vi "Signal List Keys.vi"(8 "error in":errorcluster, 11 "PRM in":refnum<class "PRM.lvclass">) -> (0 "error out":errorcluster, 2 "CFG Signal Headers":string[](array[string]), 3 "PRM out":refnum<class "PRM.lvclass">)   [LabVIEW 2019, in "PRM.lvlib" / "PRM.lvclass"]
uses:
  Library/PRM.lvclass
  Custom Controls/Signal List Keys.ctl
  builds/Instruments/Instruments.lvlibp/Library/Instruments.lvclass
panel:
  in  "Signal List Keys":T1
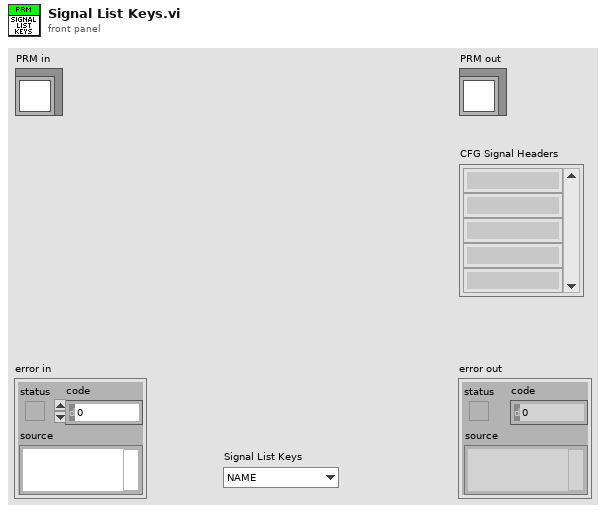
[diagram p1: front panel]
types:
  T1 = typedef "PRM.lvlib/PRM.lvclass/Signal List Keys.ctl" = enum16{"NAME", "MAX", "MIN", "RTD_A", "RTD_B", "RTD_C", "RTD_R0"}
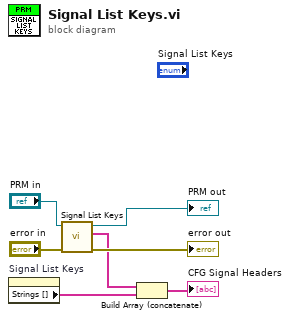
[diagram p0: block diagram]
diagram:
  n1 = property on="Signal List Keys" class="Enum (strict)"() -> ("Strings []"=w3:string[])  [unwired: 2 in, 2 out]
  n2 = call-parent "Signal List Keys.vi"("error in"="error in", "Instruments in"="PRM in") -> ("error out"=→"error out":errorcluster, "CFG Signal Headers"=w2:string[], "Instruments out"=→"PRM out":refnum<class "PRM.lvclass">)  [unwired: 7 in]
  n3 = Build Array (concatenate)(w2, w3) -> (→"CFG Signal Headers":string[])
